vi "IBM4_Read(I1).vi"(8 "error in":errorcluster, 10 "Channel":i32, 11 "COM resource in":refnum<visa-resource-name>="COM9") -> (0 "error out":errorcluster, 2 "output":i32, 3 "COM resource out":refnum<visa-resource-name>)   [LabVIEW 2021, in "IBM4.lvlib"]
uses:
  <vilib>/Instr/_visa.llb/VISA Configure Serial Port (Instr).vi
  IBM4.lvlib
panel:
  out "read buffer":string
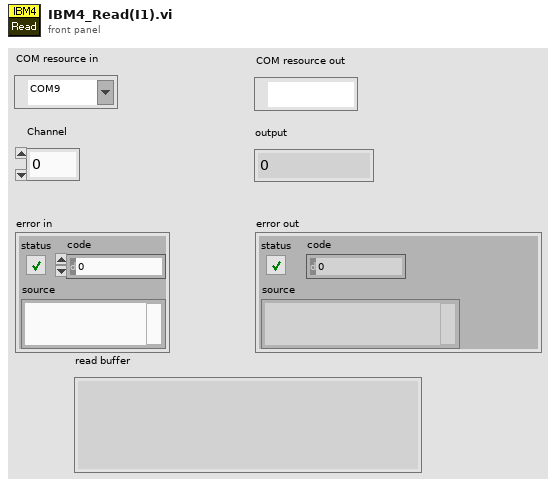
[diagram p1: front panel]
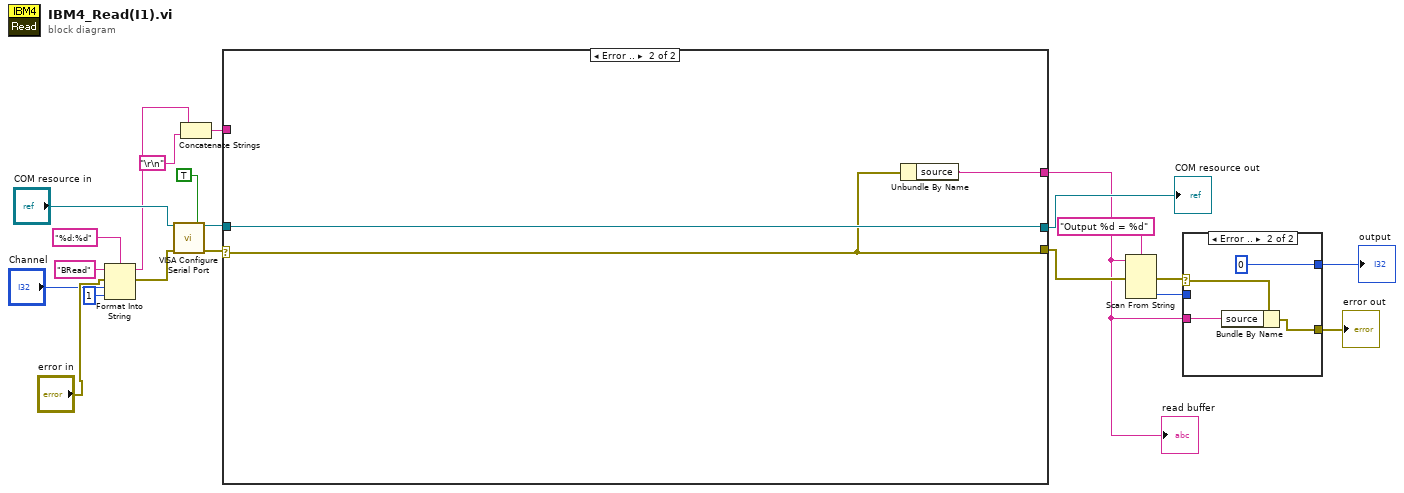
[diagram p0: block diagram]
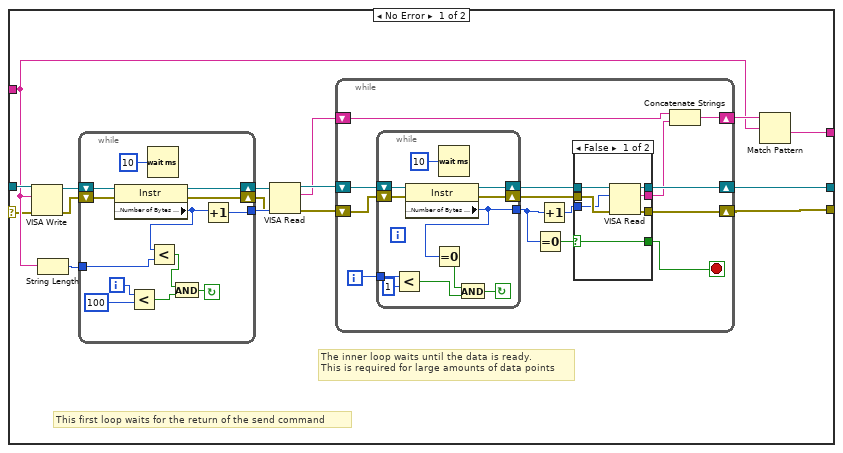
[diagram p3: hidden frame]
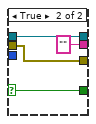
[diagram p4: hidden frame]
diagram:
  n1 = Format Into String(format string="%d:%d", initial string="BRead", error in="error in", "Channel", 1 ("input 2")) -> (resulting string=w7:string, error out=w16:errorcluster)
  n2 = call-poly "VISA Configure Serial Port"("VISA resource name"="COM resource in", "Enable Termination\nChar (T)"=TRUE ("Enable Termination\nChar (T)"), "error in (no error)"=w16) -> ("VISA resource name out"=w13:refnum<visa-resource-name>, "error out"=w12:errorcluster)  [unwired: 11 in]
  n3 = Concatenate Strings(w7, "\r\n") -> (w6:string)
  n4 = case shown="Error .." w12 {
    selector: w12 -> [w24 w87]
    tunnel: w13 -> [w37 w89]
    tunnel: [w23 w87] -> w10
    tunnel: [w35 w88] -> w1
    tunnel: w6 -> [w34 _]
    tunnel: [w22 w89] -> w11
    frame No Error {
      # "The inner loop waits until the data is ready.\nThis is required for large amounts of data points"
      # "This first loop waits for the return of the send command"
      n5 = VISA Write(VISA resource name=w37, write buffer=w34, error in (no error)=w24) -> (VISA resource name out=w33:refnum<visa-resource-name>, error out=w32:errorcluster)  [unwired: 1 out]
      n6 = String Length(string=w34) -> (length=w25:i32)
      n7 = while {
        tunnel: [w39] -> w30
        shift-right: [w49] -> w31
        shift-left: w33 -> [w50]
        shift-right: [w47] -> w29
        shift-left: w32 -> [w48]
        tunnel: w25 -> [w45]
        i -> [w40]
        stop <- w43 continue-if-true
        n8 = property class="Instr"(reference=w50, error in=w48) -> (reference out=w49:refnum<visa-resource-name>, error out=w47:errorcluster, "Serial Settings:Number of Bytes at Serial Port"=w38:u32)
        n9 = Less?(x=w40, y=100) -> (x < y?=w42:bool)
        n10 = Wait (ms)(milliseconds to wait=u32 10) -> ()  [unwired: 1 out]
        n11 = Less?(x=w38, y=w45) -> (x < y?=w41:bool)
        n12 = And(x=w41, y=w42) -> (x .and. y?=w43:bool)
        n13 = Increment(x=w38) -> (x+1=w39:u32)
      }
      n14 = VISA Read(VISA resource name=w31, byte count=w30, error in (no error)=w29) -> (VISA resource name out=w28:refnum<visa-resource-name>, read buffer=w26:string, error out=w27:errorcluster)  [unwired: 1 out]
      n15 = while {
        shift-right: [w64] -> w22
        shift-left: w28 -> [w62]
        shift-right: [w63] -> w23
        shift-left: w27 -> [w60]
        shift-right: [w58] -> w36
        shift-left: w26 -> [w56]
        i -> [w55]
        stop <- w51 stop-if-true
        n16 = while {
          tunnel: [w81] -> w54
          shift-right: [w85] -> w61
          shift-left: w62 -> [w86]
          shift-right: [w83] -> w59
          shift-left: w60 -> [w84]
          tunnel: w55 -> [w80]
          stop <- w78 continue-if-true
          n17 = Less?(x=w80, y=1) -> (x < y?=w77:bool)
          n18 = property class="Instr"(reference=w86, error in=w84) -> (reference out=w85:refnum<visa-resource-name>, error out=w83:errorcluster, "Serial Settings:Number of Bytes at Serial Port"=w81:u32)
          n19 = Equal To 0?(x=w81) -> (x = 0?=w76:bool)
          n20 = Wait (ms)(milliseconds to wait=u32 10) -> ()  [unwired: 1 out]
          n21 = And(x=w76, y=w77) -> (x .and. y?=w78:bool)
        }
        n22 = Equal To 0?(x=w54) -> (x = 0?=w52:bool)
        n23 = Increment(x=w54) -> (x+1=w53:u32)
        n24 = case shown="False" w52 {
          selector: w52 -> [w65 w74]
          tunnel: [w71 w75] -> w64
          tunnel: [w70 w73] -> w63
          tunnel: w61 -> [w69 w75]
          tunnel: w59 -> [w68 w73]
          tunnel: [w67 "" ("read buffer")] -> w57
          tunnel: w53 -> [w66 _]
          tunnel: [w65 w74] -> w51
          frame False {
            n25 = VISA Read(VISA resource name=w69, byte count=w66, error in (no error)=w68) -> (VISA resource name out=w71:refnum<visa-resource-name>, read buffer=w67:string, error out=w70:errorcluster)  [unwired: 1 out]
          }
          frame True {
          }
        }
        n26 = Concatenate Strings(w56, w57) -> (w58:string)
      }
      n27 = Match Pattern(string=w36, regular expression=w34) -> (after substring=w35:string)  [unwired: 1 in, 3 out]
    }
    frame Error {
      n28 = Unbundle By Name(w87) -> ("source"=w88:string)
    }
  }
  "COM resource out" <- w11
  "read buffer" <- w1
  n29 = Scan From String(format string="Output %d = %d", input string=w1, error in=w10) -> (error out=w5:errorcluster, output 2=w4:i32)  [unwired: 4 in, 2 out]
  n30 = case shown="Error .." w5 {
    selector: w5 -> [w90 w94]
    tunnel: w4 -> [w91 _]
    tunnel: [w91 0] -> w3
    tunnel: [w90 w92] -> w2
    tunnel: w1 -> [_ w93]
    frame No Error {
    }
    frame Error {
      n31 = Bundle By Name(cluster=w94, "source"=w93) -> (w92:errorcluster)
    }
  }
  "error out" <- w2
  "output" <- w3
